vi "load_config_essai.vi"() -> ()   [LabVIEW 2013]
uses:
  <vilib>/Analysis/Matrix/Datatypes/RealMatrix.ctl
  <vilib>/Analysis/Matrix/NI_Matrix.lvlib
panel:
  out "USED_FILTERS":u8[](array[numeric])
  out "USED_LEDS":bool[][](array[boolean])
  out "Nstart":u32=30 step=1
  out "Non":u32=150 step=1
  out "Noff":u32 step=1
  out "BETWEEN_PAT":u32
  out "NPAT":u32
  out "BETWEEN_SCAN":u32
  out "NSCAN":u32
  out "XYPOS":T1
  out "STAGE_PORT":refnum<visa-resource-name>="COM1"
  out "STAGE_SPEED":dbl
  out "ROMODE":u32
  out "BIN":u16
  out "EXPT":dbl
  in  "Config Directory":path=path "D:/ParDates"
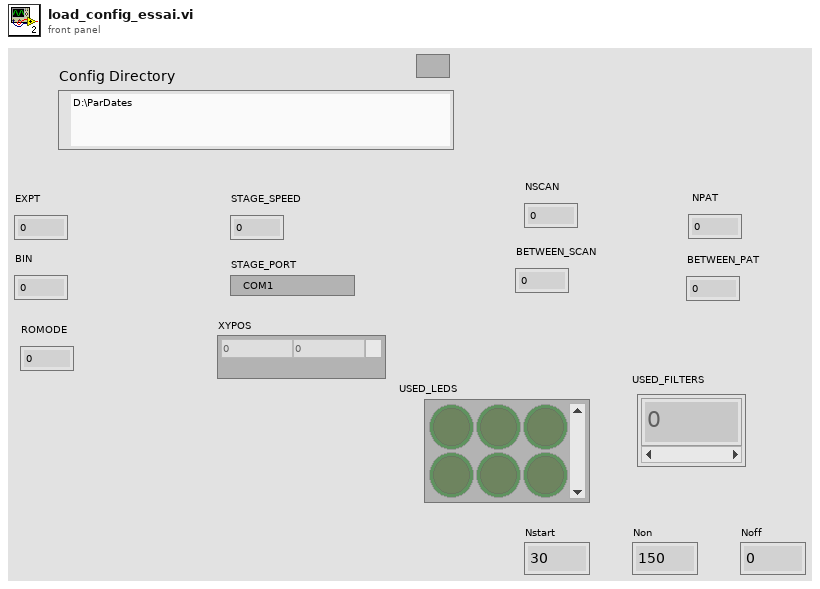
[diagram p1: front panel]
types:
  T1 = typedef "NI_Matrix.lvlib/RealMatrix.ctl" = dbl[][]
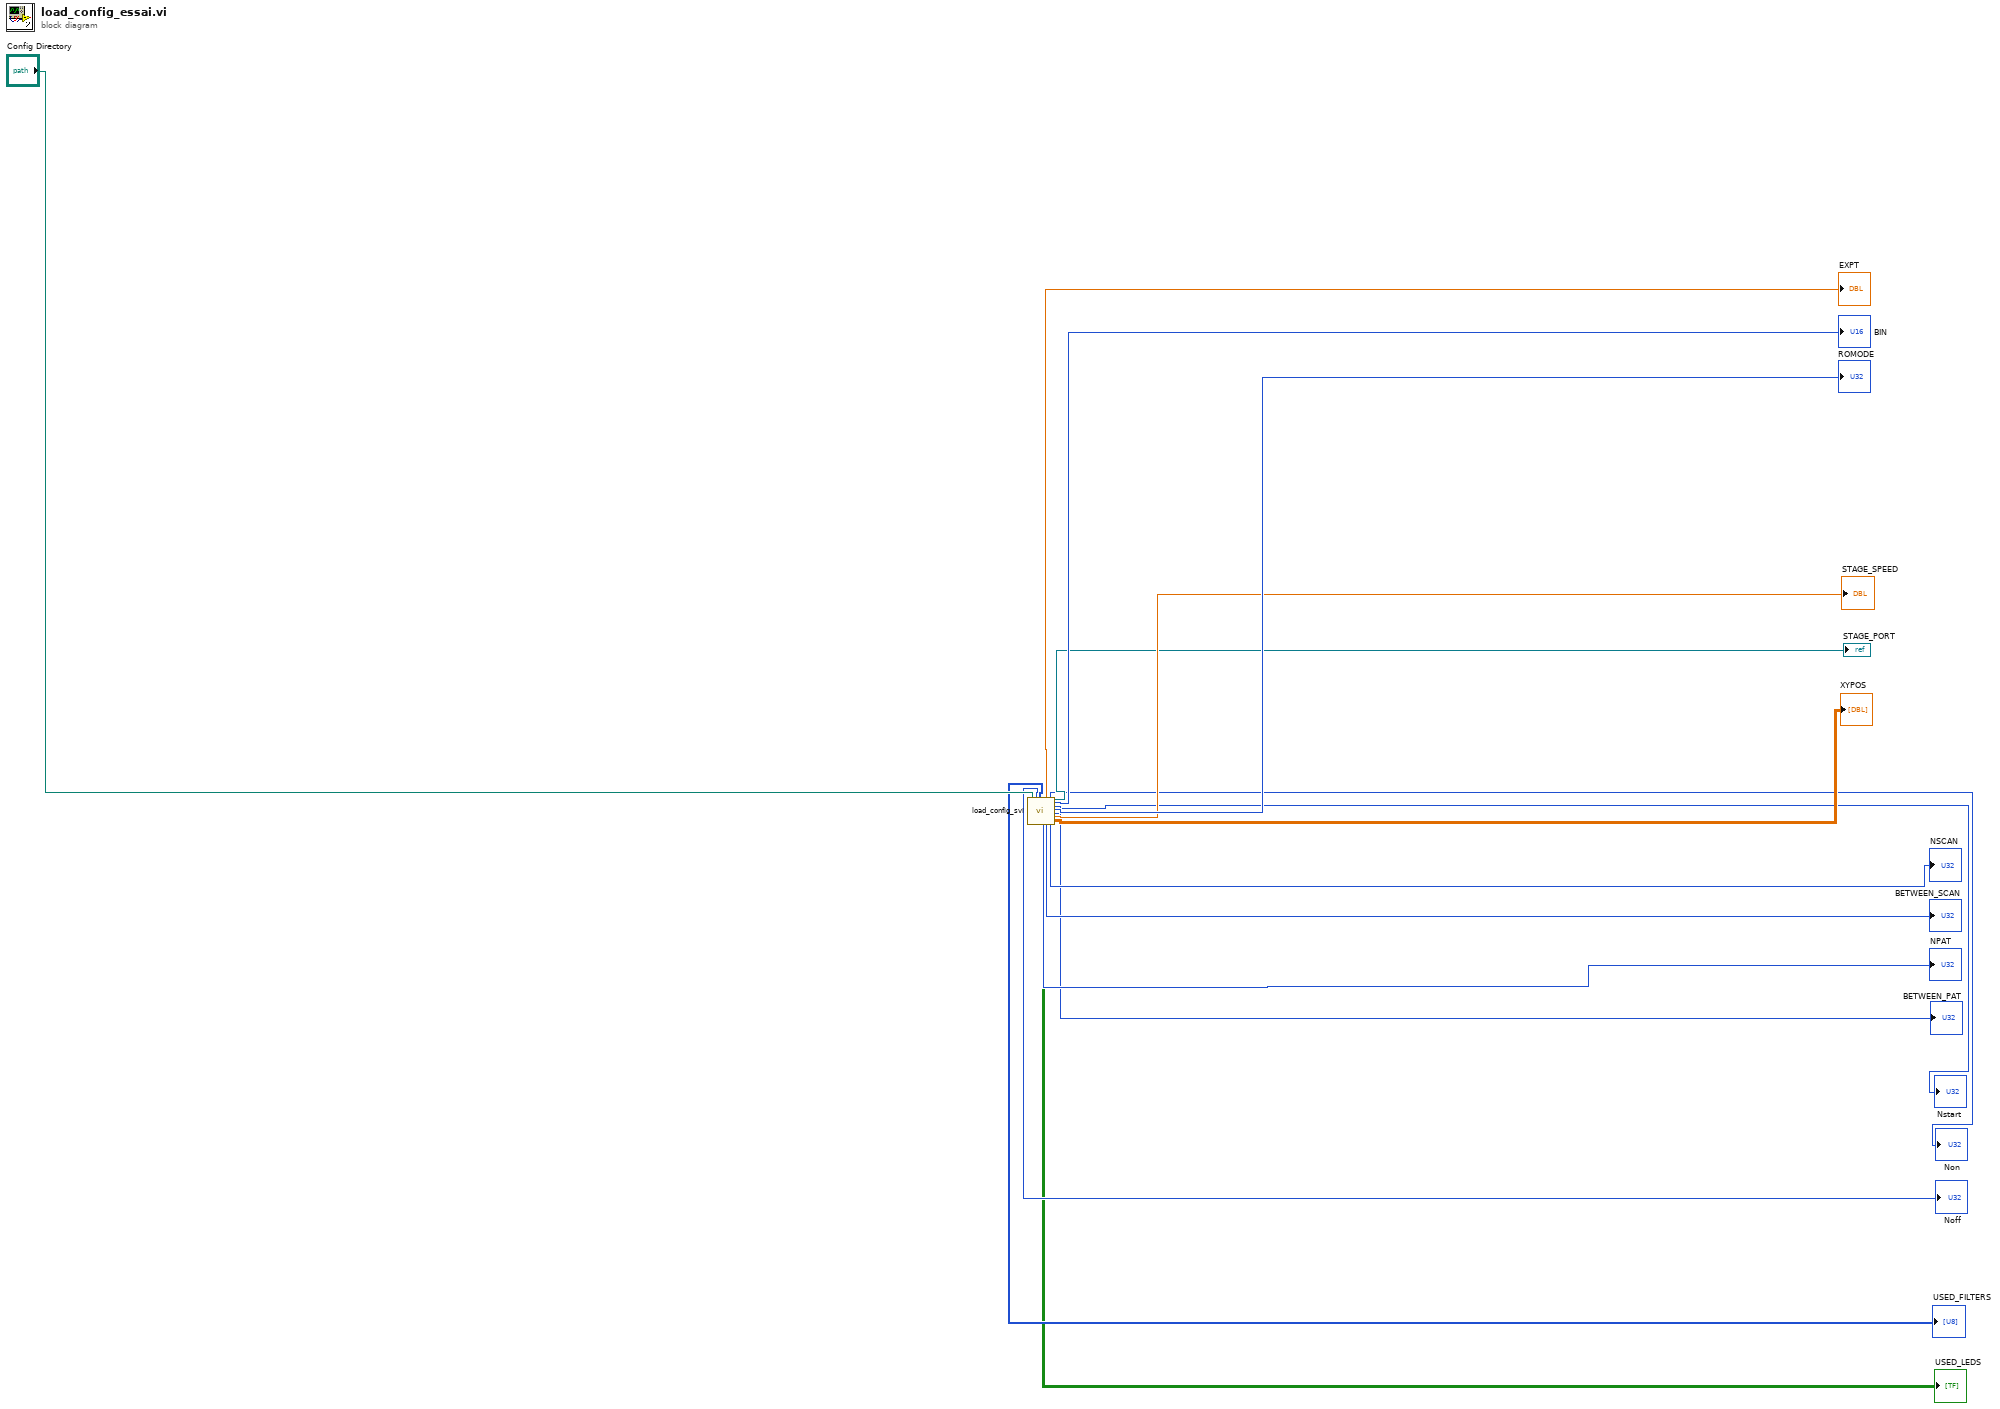
[diagram p0: block diagram]
diagram:
  n1 = call "load_config_svi.vi"("Config Directory"="Config Directory") -> ("Noff"=→"Noff":u32, "USED_FILTERS"=→"USED_FILTERS":u8[], "USED_LEDS"=→"USED_LEDS":bool[][], "NPAT"=→"NPAT":u32, "EXPT"=→"EXPT":dbl, "BETWEEN_SCAN"=→"BETWEEN_SCAN":u32, "Non"=→"Non":u32, "NSCAN"=→"NSCAN":u32, "Refnum VISA en sortie"=→"STAGE_PORT":refnum<visa-resource-name>, "BIN"=→"BIN":u16, "Nstart"=→"Nstart":u32, "ROMODE"=→"ROMODE":u32, "BETWEEN_PAT"=→"BETWEEN_PAT":u32, "STAGE_SPEED"=→"STAGE_SPEED":dbl, "XYPOS"=→"XYPOS":T1)  [unwired: 12 in]
